vi "AK SATK FGV.vi"(6 "Aktion":T1, 11 "Cluster (in)":cluster{"SATK":bool}) -> (3 "Cluster (out)":cluster{"SATK":bool})   [LabVIEW 2020, in "AK-Schnittstelle.lvlib"]
uses:
  AK SATK Aktion.ctl
  AK-Schnittstelle.lvlib
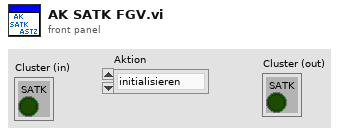
[diagram p1: front panel]
types:
  T1 = typedef "AK-Schnittstelle.lvlib/AK SATK Aktion.ctl" = enum16{"initialisieren", "lesen", "schreiben"}
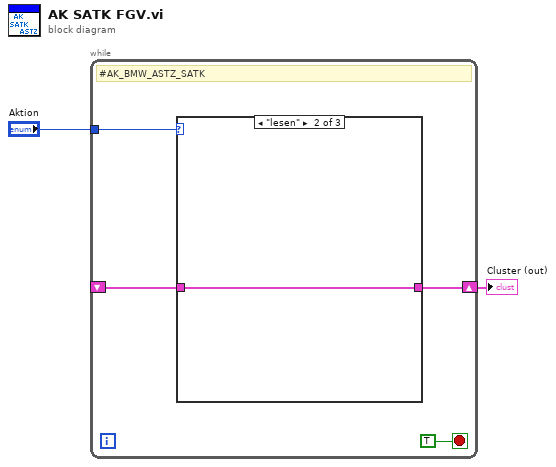
[diagram p0: block diagram]
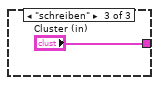
[diagram p3: hidden frame]
diagram:
  n1 = while {
    tunnel: "Aktion" -> [w5]
    shift-right: [w4] -> w1
    shift-left: _ -> [w3]
    stop <- TRUE stop-if-true
    # "#AK_BMW_ASTZ_SATK"
    n2 = case shown="\"lesen\"" w5 {
      tunnel: [_ w7 "Cluster (in)"] -> w4
      tunnel: w3 -> [_ w7 _]
      frame "initialisieren", Default {
      }
      frame "lesen" {
      }
      frame "schreiben" {
      }
    }
  }
  "Cluster (out)" <- w1
